vi "New Gate Sweep.vi"() -> ()   [LabVIEW 2010]
panel:
  out "Gate voltage(V)":string
  in  "Channel":dbl
  in  "Number of Avg":dbl
  in  "Bias":dbl
  out "Sweep Time (s)":string
  in  "End Settling Time":dbl
  in  "Max Gate Slew Rate (V/s)":dbl
  in  "Z Averaging Time":dbl
  in  "Integration Time":dbl
  in  "Settling Time":dbl
  out "Points":string
  in  "Initial Settling Time":dbl
  in  "Step Size(V)":dbl
  in  "End Gate (V)":dbl
  in  "Start Gate (V)":dbl
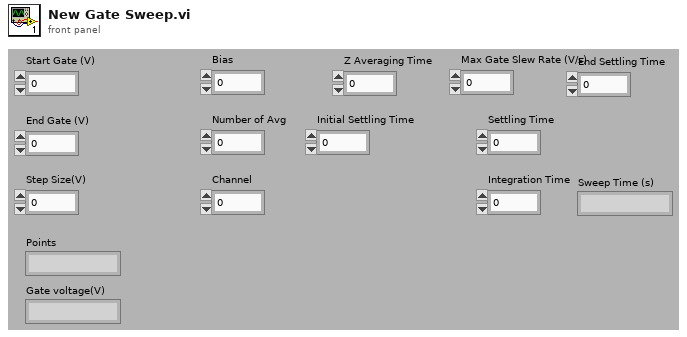
[diagram p1: front panel]
types:
  T1 = enum16{"Set Voltage", "Read Voltage", "Read Setpoint", "Read Current", "Output On", "Output Off"}
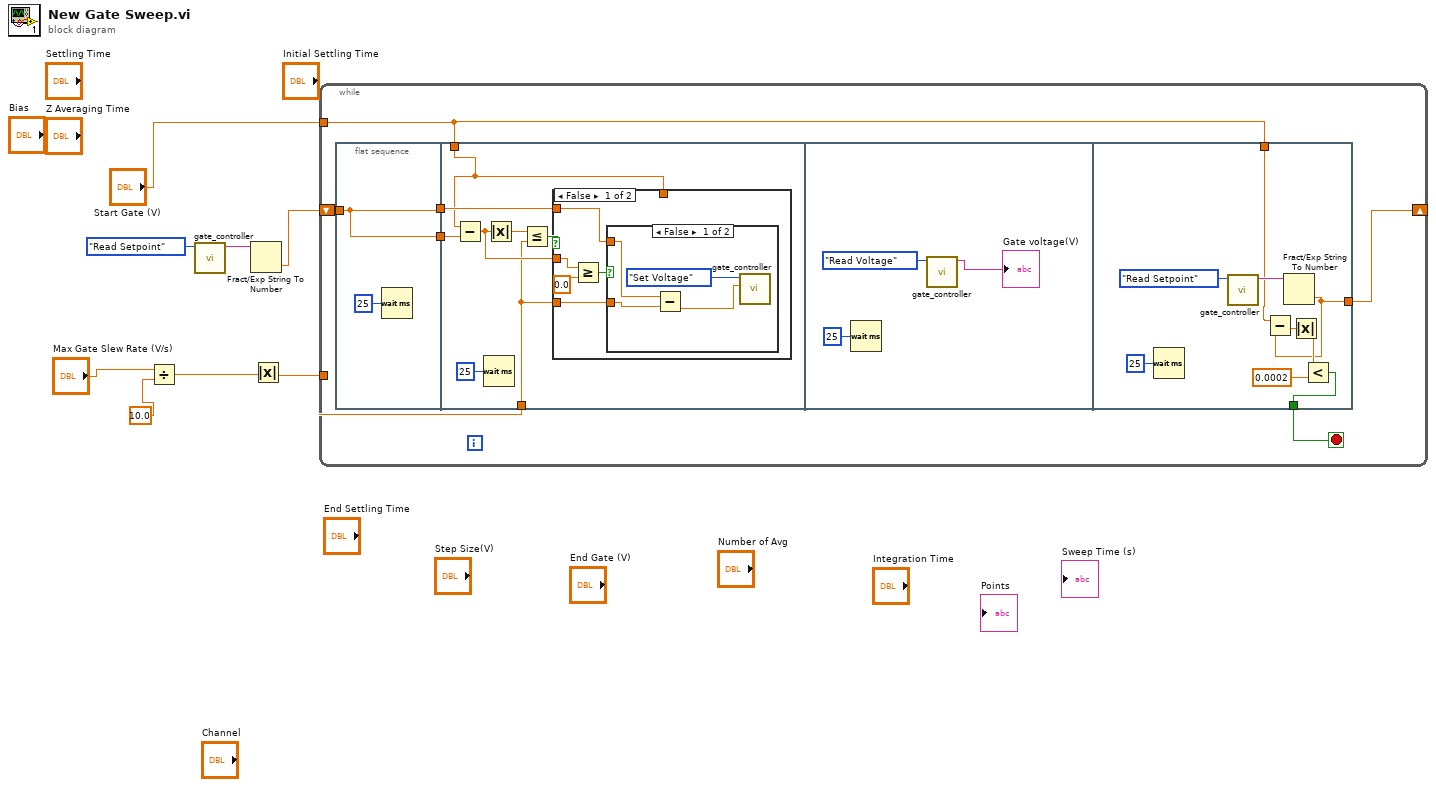
[diagram p0: block diagram]
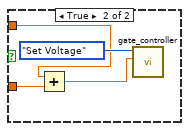
[diagram p2: hidden frame]
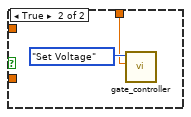
[diagram p3: hidden frame]
diagram:
  n1 = Divide(x="Max Gate Slew Rate (V/s)", y=10.0) -> (x/y=w1:dbl)
  n2 = call "gate_controller.vi"("Command"=T1."Read Setpoint") -> ("Response"=w8:string)  [unwired: 10 in]
  n3 = Fract/Exp String To Number(string=w8) -> (number=w6:dbl)  [unwired: 3 in, 1 out]
  n4 = Absolute Value(x=w1) -> (abs(x)=w5:dbl)
  n5 = while {
    tunnel: w5 -> [w14]
    shift-right: [w10] -> _
    shift-left: w6 -> [w11]
    tunnel: "Start Gate (V)" -> [w9]
    stop <- w13 stop-if-true
    n6 = flat-sequence {
      tunnel: [w16] -> w15
      tunnel: [w16] -> w12
      tunnel: w11 -> [w16]
      tunnel: w9 -> [w18]
      tunnel: w15 -> [w25]
      tunnel: w14 -> [w20]
      tunnel: w12 -> [w19]
      tunnel: w9 -> [w49]
      tunnel: [w45] -> w13
      tunnel: [w44] -> w10
      frame #0 {
        n7 = Wait (ms)(milliseconds to wait=u32 25) -> ()  [unwired: 1 out]
      }
      frame #1 {
        n8 = Subtract(x=w18, y=w25) -> (x-y=w21:dbl)
        n9 = Wait (ms)(milliseconds to wait=u32 25) -> ()  [unwired: 1 out]
        n10 = Absolute Value(x=w21) -> (abs(x)=w24:dbl)
        n11 = Less Or Equal?(x=w24, y=w20) -> (x <= y?=w23:bool)
        n12 = case shown="False" w23 {
          tunnel: w18 -> [_ w39]
          tunnel: w21 -> [w27 _]
          tunnel: w20 -> [w30 _]
          tunnel: w19 -> [w26 _]
          frame False {
            n13 = Greater Or Equal?(x=w27, y=0.0) -> (x >= y?=w29:bool)
            n14 = case shown="False" w29 {
              tunnel: w30 -> [w32 w37]
              tunnel: w26 -> [w31 w35]
              frame False {
                n15 = Subtract(x=w31, y=w32) -> (x-y=w33:dbl)
                n16 = call "gate_controller.vi"("Numerical Argument"=w33, "Command"=T1."Set Voltage") -> ()  [unwired: 9 in, 1 out]
              }
              frame True {
                n17 = Add(x=w35, y=w37) -> (x+y=w36:dbl)
                n18 = call "gate_controller.vi"("Numerical Argument"=w36, "Command"=T1."Set Voltage") -> ()  [unwired: 9 in, 1 out]
              }
            }
          }
          frame True {
            n19 = call "gate_controller.vi"("Numerical Argument"=w39, "Command"=T1."Set Voltage") -> ()  [unwired: 9 in, 1 out]
          }
        }
      }
      frame #2 {
        n20 = Wait (ms)(milliseconds to wait=u32 25) -> ()  [unwired: 1 out]
        n21 = call "gate_controller.vi"("Command"=T1."Read Voltage") -> ("Response"=→"Gate voltage(V)":string)  [unwired: 10 in]
      }
      frame #3 {
        n22 = Wait (ms)(milliseconds to wait=u32 25) -> ()  [unwired: 1 out]
        n23 = call "gate_controller.vi"("Command"=T1."Read Setpoint") -> ("Response"=w51:string)  [unwired: 10 in]
        n24 = Fract/Exp String To Number(string=w51) -> (number=w44:dbl)  [unwired: 3 in, 1 out]
        n25 = Subtract(x=w49, y=w44) -> (x-y=w48:dbl)
        n26 = Absolute Value(x=w48) -> (abs(x)=w47:dbl)
        n27 = Less?(x=w47, y=0.0002) -> (x < y?=w45:bool)
      }
    }
  }
